vi "Cycle.vi"(8 "error in (no error)":errorcluster, 11 "DotMapping.lvclass":refnum<class "DotMapping.lvclass">) -> (0 "error out":errorcluster, 3 "DotMapping.lvclass 2":refnum<class "DotMapping.lvclass">)   [LabVIEW 2010, in "DotMapping.lvclass"]
uses:
  DotMapping.lvclass
  PassiveExperiment/PassiveExperiment.lvclass
panel:
  out "Timeouts":T1={"Intertrial"=1000.0, "AcquireFixation"=1000.0, "HoldFixation"=300.0, "DelayPeriod"=1000.0, "ResponsePeriod"=1000.0}
  out "ExperimentStats":T2
  out "Cycles":dbl
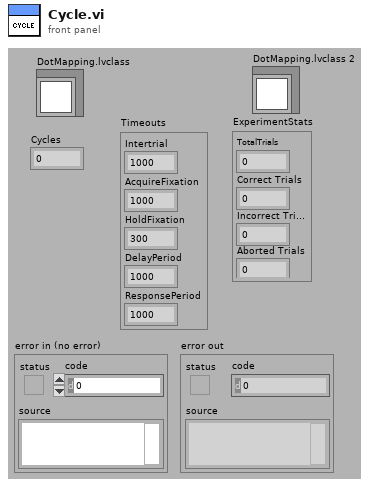
[diagram p1: front panel]
types:
  T1 = cluster{"Intertrial":dbl, "AcquireFixation":dbl, "HoldFixation":dbl, "DelayPeriod":dbl, "ResponsePeriod":dbl}
  T2 = cluster{"TotalTrials":dbl, "Correct Trials":dbl, "Incorrect Trials":dbl, "Aborted Trials":dbl}
  T3 = cluster{"TotalTrials":u32, "Correct Trials":u32, "Incorrect Trials":u32, "Aborted Trials":u32}
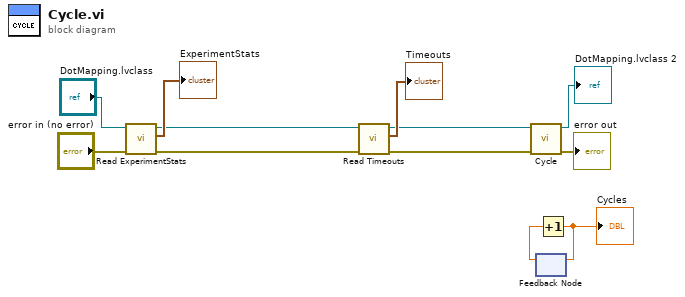
[diagram p0: block diagram]
diagram:
  n1 = call-dynamic "Read ExperimentStats.vi"("error in (no error)"="error in (no error)", "TrialBasedExperiment in"="DotMapping.lvclass") -> ("error out"=w6:errorcluster, "ExperimentStats"=→"ExperimentStats":T3, "TrialBasedExperiment out"=w7:refnum<class "DotMapping.lvclass">)  [unwired: 7 in]
  n2 = call-dynamic "Read Timeouts.vi"("error in (no error)"=w6, "TrialBasedExperiment in"=w7) -> ("error out"=w5:errorcluster, "Timeouts"=→"Timeouts":T1, "TrialBasedExperiment out"=w3:refnum<class "DotMapping.lvclass">)  [unwired: 7 in]
  n3 = call-parent "Cycle.vi"("error in (no error)"=w5, "PassiveExperiment In"=w3) -> ("error out"=→"error out":errorcluster, "PassiveExperiment Out"=→"DotMapping.lvclass 2":refnum<class "DotMapping.lvclass">)  [unwired: 8 in]
  n4 = feedback #1() -> (w10:dbl)  [unwired: 1 in]
  n5 = Increment(x=w10) -> (x+1=w11:dbl)
  "Cycles" <- w11
  n6 = feedback-in #1(w11) -> ()
